vi "Set state dt (t).vi"(8 "Error In":errorcluster, 10 "dt (ms)":u32, 11 "VISA resource name in":refnum<visa-resource-name>) -> (0 "Error out":errorcluster, 1 "ACK":bool, 3 "VISA resource name out":refnum<visa-resource-name>)   [LabVIEW 2020]
uses:
  Ctls/Cmd str.ctl
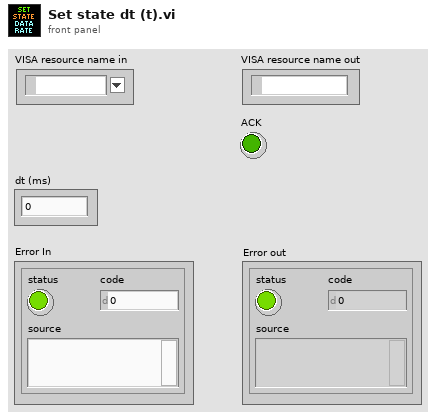
[diagram p1: front panel]
types:
  T1 = typedef "Cmd str.ctl" = string
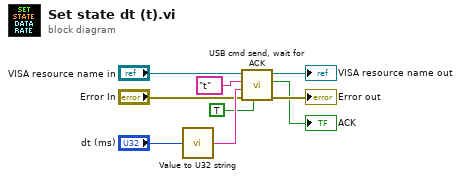
[diagram p0: block diagram]
diagram:
  n1 = call "Value to U32 string.vi"("Value"="dt (ms)") -> ("U32 str (Little Endian)"=w9:string)
  n2 = call "USB cmd send, wait for ACK.vi"("Wait for ACK?"=TRUE, "Error In"="Error In", "4 byte config str"=w9, "Cmd"=T1 "t", "VISA resource name in"="VISA resource name in") -> ("Error out"=→"Error out":errorcluster, "ACK ok"=→"ACK":bool, "VISA resource name out"=→"VISA resource name out":refnum<visa-resource-name>)  [unwired: 1 in, 1 out]
